vi "LineDetect.vi"(7 "Mode":T2, 9 "NXT In":T3) -> (1 "Line Found?":bool, 3 "NXT Out":T3)   [LabVIEW 2012]
uses:
  <vilib>/NXT/Subs/LVHSConnector.ctl
  <vilib>/NXT/LegoClasses/BrickReference/BrickReference.lvclass
  LineDetectCtl.ctl
  <vilib>/NXT/Block Support/NXT_InputPort.ctl
  LiteDifferControl.ctl
  <vilib>/NXT/Dual Mode Library/Sensors/Light_On.vi
panel:
  in  "Port (Port 3)":T1=2 items=["Port 1", "Port 2", "Port 3", "Port 4"]
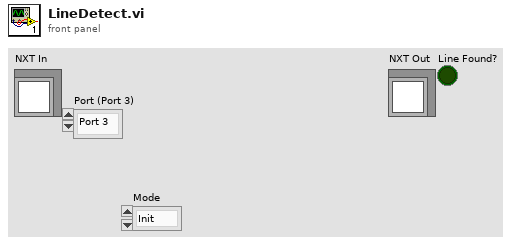
[diagram p1: front panel]
types:
  T1 = typedef "NXT_InputPort.ctl" = u8
  T2 = typedef "LineDetectCtl.ctl" = enum16{"Init", "Found?", "Close"}
  T3 = typedef "LVHSConnector.ctl" = refnum<class "BrickReference.lvclass">
  T4 = typedef "LiteDifferControl.ctl" = enum16{"Less", "Greater"}
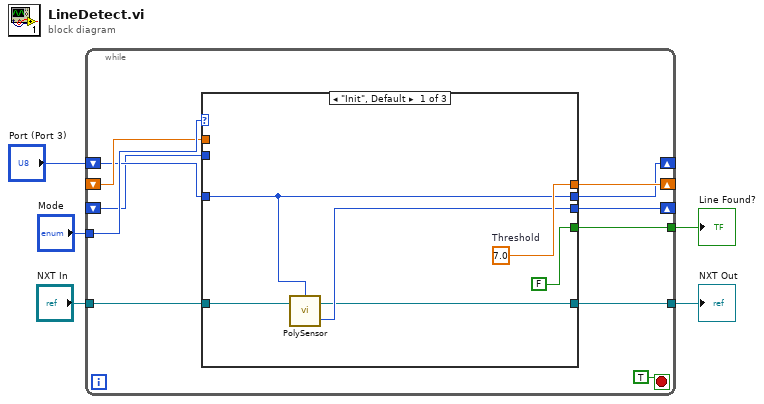
[diagram p0: block diagram]
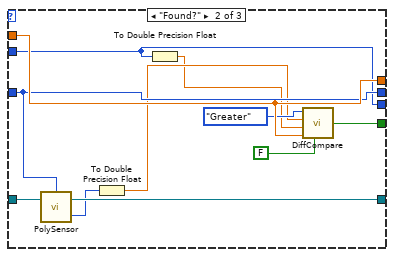
[diagram p2: hidden frame]
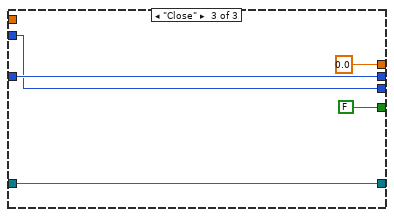
[diagram p3: hidden frame]
diagram:
  n1 = while {
    tunnel: "Mode" -> [w15]
    tunnel: "NXT In" -> [w14]
    tunnel: [w13] -> w4
    shift-right: [w12] -> _
    shift-left: _ -> [w11]
    tunnel: [w10] -> w2
    shift-right: [w8] -> _
    shift-left: "Port (Port 3)" -> [w9]
    shift-right: [w7] -> _
    shift-left: _ -> [w6]
    stop <- TRUE stop-if-true
    n2 = case shown="\"Init\", Default" w15 {
      tunnel: w14 -> [w18 w29 w37]
      tunnel: [w17 w28 w37] -> w13
      tunnel: [w21 w33 0.0] -> w12
      tunnel: w11 -> [_ w33 _]
      tunnel: [FALSE ("Result") w31 FALSE ("Result")] -> w10
      tunnel: w9 -> [w19 w27 w35]
      tunnel: [w19 w27 w35] -> w8
      tunnel: w6 -> [_ w24 w34]
      tunnel: [w20 w24 w34] -> w7
      frame "Init", Default {
        w21 = 7.0  # Threshold
        n3 = call-poly <vilib>:"PolySensor.vi"("NXT"=w18, "Port (Port 3)"=w19) -> ("Scaled Value"=w20:i16, "NXT"=w17:T3)  [unwired: 1 in]
      }
      frame "Found?" {
        n4 = call-poly <vilib>:"PolySensor.vi"("NXT"=w29, "Port (Port 3)"=w27) -> ("Scaled Value"=w26:i16, "NXT"=w28:T3)  [unwired: 1 in]
        n5 = To Double Precision Float(number=w26) -> (double precision float=w25:dbl)
        n6 = To Double Precision Float(number=w24) -> (double precision float=w23:dbl)
        n7 = call "DiffCompare.vi"("Comparison"=LiteDifferControl."Greater", "X"=w25, "Y"=w23, "Absolute Diff?"=FALSE, "Threshold"=w33) -> ("Result"=w31:bool)  [unwired: 3 in]
      }
      frame "Close" {
      }
    }
  }
  "NXT Out" <- w4
  "Line Found?" <- w2
